vi "testdelay.vi"(8 "error in (no error)":errorcluster, 11 "Application ref in":refnum<vi>) -> (0 "error out":errorcluster, 2 "Boolean":bool=TRUE, 3 "Application ref out":refnum<vi>)   [LabVIEW 2017]
uses:
  <userlib>/Nanonis Prog Interface V5/Nanonis Prog Interface.lvlib
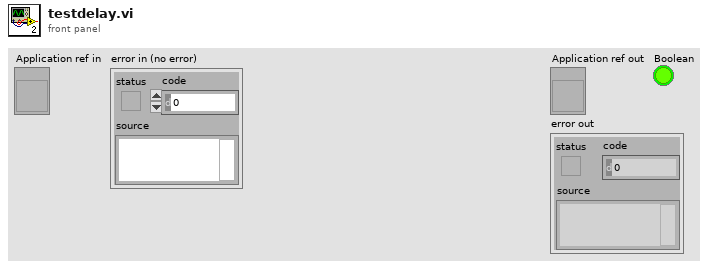
[diagram p1: front panel]
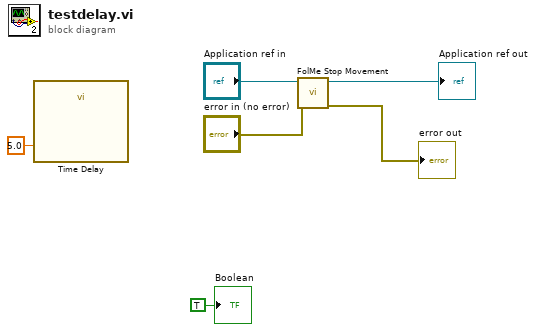
[diagram p0: block diagram]
diagram:
  n1 = call "Time Delay"("Delay Time (s)"=5.0) -> ()  [unwired: 10 in, 1 out]
  n2 = call <userlib>:"FolMe Stop Movement.vi"("error in (no error)"="error in (no error)", "Application ref in"="Application ref in") -> ("error out"=→"error out":errorcluster, "Application ref out"=→"Application ref out":refnum<vi>)  [unwired: 6 in]
  "Boolean" <- TRUE
